vi "Generate AO Sweep Waveforms.vi"(8 "error in (no error)":errorcluster, 11 "Generator":refnum<class "Generator.lvclass">) -> (0 "error out":errorcluster, 2 "AO Array":waveform(dbl)[](array[waveform]), 3 "Generator out":refnum<class "Generator.lvclass">)   [LabVIEW 2019, in "Generator.lvclass"]
uses:
  Generator.lvclass
  typedefs/Generator.Sweep Status--enum.ctl
  typedefs/Generator.Sweep State--enum.ctl
  Generator.lvclass/Generator.ctl
  Waveform.Attributes/Waveform.Attributes.lvlib
panel:
  in  "Tab Control":enum32{"Page 1", "Graphs"}(tab)
  out "Waveform Graph":waveform(dbl)[](graph)
  out "sweep status":T1
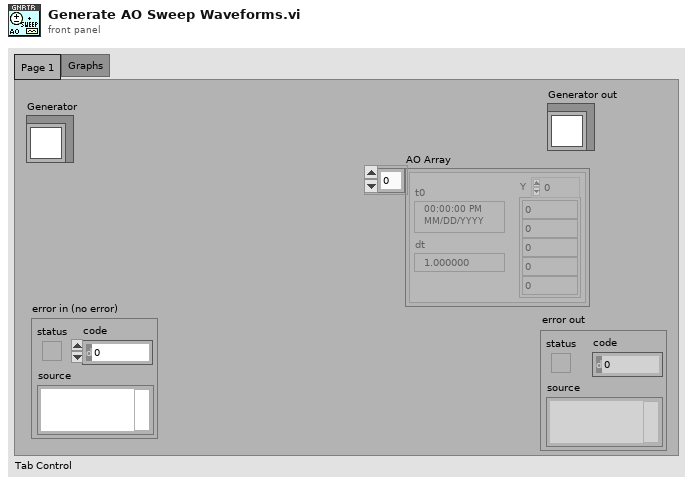
[diagram p1: front panel]
types:
  T1 = typedef "Generator.lvclass/Generator.Sweep Status--enum.ctl" = enum16{"idle", "initializing", "waiting", "sweeping", "stopping"}
  T2 = typedef "Generator.lvclass/Generator.Sweep State--enum.ctl" = enum16{"idle", "initialize", "wait", "sweep", "stop"}
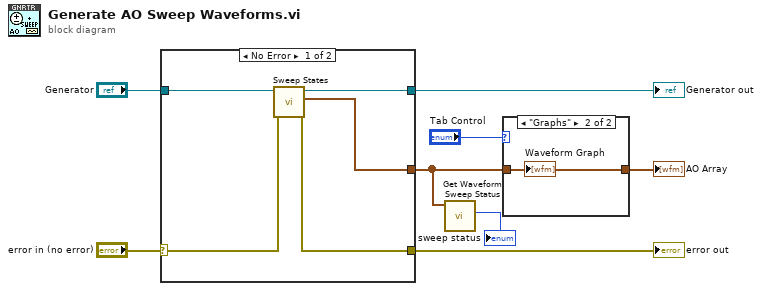
[diagram p0: block diagram]
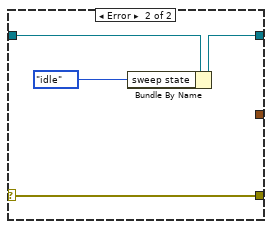
[diagram p2: hidden frame]
diagram:
  n1 = case shown="No Error" "error in (no error)" {
    selector: "error in (no error)" -> [w10 w17]
    tunnel: "Generator" -> [w13 w14]
    tunnel: [w12 w15] -> w7
    tunnel: [w11 w17] -> w6
    tunnel: [w9 _] -> w2
    frame No Error {
      n2 = call "Sweep States.vi"("error in (no error)"=w10, "Generator in"=w13) -> ("error out"=w11:errorcluster, "Waveforms out"=w9:waveform(dbl)[], "Generator out"=w12:refnum<class "Generator.lvclass">)  [unwired: 7 in]
    }
    frame Error {
      n3 = Bundle By Name(cluster=w14, "sweep state"=Generator.Sweep_State--enum."idle" ("sweep state out")) -> (w15:refnum<class "Generator.lvclass">)
    }
  }
  "error out" <- w6
  "Generator out" <- w7
  n4 = call "Get Waveform Sweep Status.vi"("Waveforms in"=w2) -> ("sweep status"=→"sweep status":T1)  [unwired: 8 in, 2 out]
  n5 = case shown="\"Graphs\"" "Tab Control" {
    tunnel: w2 -> [w18 w19]
    tunnel: [w18 w19] -> w3
    frame Default {
    }
    frame "Graphs" {
      "Waveform Graph" <- w19
    }
  }
  "AO Array" <- w3
